vi "BurstAcel.vi"(8 "error in":errorcluster, 11 "acelData":dbl[][](array[numeric])) -> (0 "error out":errorcluster)   [LabVIEW 2016]
uses:
  MainFGV_mods.ctl
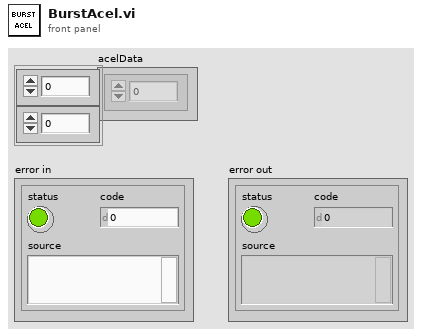
[diagram p1: front panel]
types:
  T1 = typedef "MainFGV_mods.ctl" = enum16{"Init", "Config", "Advanced", "CreateTask", "Register", "Acquire", "Start", "Burst", "Record", "End"}
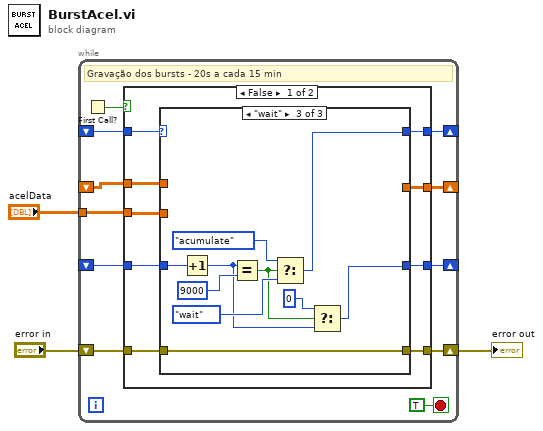
[diagram p0: block diagram]
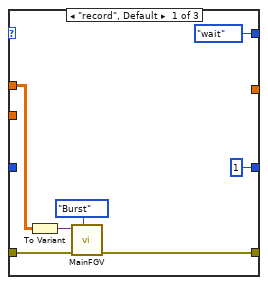
[diagram p2: hidden frame]
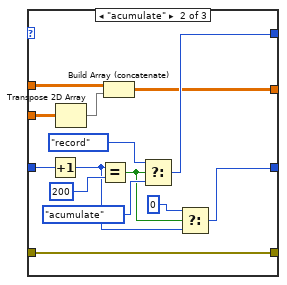
[diagram p3: hidden frame]
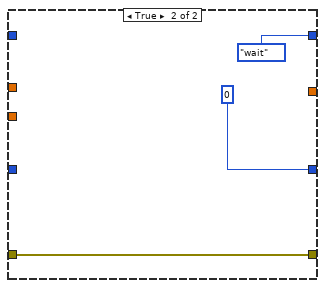
[diagram p4: hidden frame]
diagram:
  n1 = while {
    shift-right: [w13] -> _
    shift-left: _ -> [w12]
    shift-right: [w9] -> w3
    shift-left: "error in" -> [w11]
    tunnel: "acelData" -> [w10]
    shift-right: [w8] -> _
    shift-left: _ -> [w7]
    shift-right: [w5] -> _
    shift-left: _ -> [w4]
    stop <- TRUE stop-if-true
    # "Gravação dos bursts - 20s a cada 15 min"
    n2 = First Call?() -> (First Call?: T/F=w6:bool)
    n3 = case shown="False" w6 {
      tunnel: [w21 0] -> w13
      tunnel: w12 -> [w23 _]
      tunnel: w11 -> [w19 w56]
      tunnel: w10 -> [w17 _]
      tunnel: [w18 w56] -> w9
      tunnel: [w20 enum16{"record", "acumulate", "wait"}."wait"] -> w8
      tunnel: w7 -> [w22 _]
      tunnel: [w16 _] -> w5
      tunnel: w4 -> [w15 _]
      frame False {
        n4 = case shown="\"wait\"" w22 {
          tunnel: w23 -> [_ w44 w54]
          tunnel: [1 ("y") w37 w47] -> w21
          tunnel: [enum16{"record", "acumulate", "wait"}."wait" w36 w46] -> w20
          tunnel: [w24 w35 w45] -> w18
          tunnel: w19 -> [w26 w35 w45]
          tunnel: w17 -> [_ w34 _]
          tunnel: [_ w32 _] -> w16
          tunnel: w15 -> [w25 w31 _]
          frame "record", Default {
            n5 = To Variant(anything=w25) -> (Variant=w27:variant)
            n6 = call "MainFGV.vi"("FGV_mods"=MainFGV_mods."Burst", "Error In"=w26, "DataIn"=w27) -> ("Error Out"=w24:errorcluster)  [unwired: 7 in, 1 out]
          }
          frame "acumulate" {
            n7 = Increment(x=w44) -> (x+1=w39:i32)
            n8 = Transpose 2D Array(2D array=w34) -> (transposed array=w33:dbl[][])
            n9 = Equal?(x=w39, y=200) -> (x = y?=w40:bool)
            n10 = Build Array (concatenate)(w31, w33) -> (w32:dbl[][])
            n11 = Select(t=enum16{"record", "acumulate", "wait"}."record", s=w40, f=enum16{"record", "acumulate", "wait"}."acumulate") -> (s? t:f=w36:enum16{"record", "acumulate", "wait"})
            n12 = Select(t=0 ("y"), s=w40, f=w39) -> (s? t:f=w37:i32)
          }
          frame "wait" {
            n13 = Increment(x=w54) -> (x+1=w49:i32)
            n14 = Equal?(x=w49, y=9000) -> (x = y?=w50:bool)
            n15 = Select(t=enum16{"record", "acumulate", "wait"}."acumulate", s=w50, f=enum16{"record", "acumulate", "wait"}."wait") -> (s? t:f=w46:enum16{"record", "acumulate", "wait"})
            n16 = Select(t=0 ("y"), s=w50, f=w49) -> (s? t:f=w47:i32)
          }
        }
      }
      frame True {
      }
    }
  }
  "error out" <- w3
